vi "Get Owning Path Default Value.vi"(0 "Vector 26GHz Path Group in":refnum<class "Vector 26GHz Path Group.lvclass">, 11 "error in (no error)":errorcluster) -> (4 "Vector 26GHz Path Group out":refnum<class "Vector 26GHz Path Group.lvclass">, 6 "Path":refnum<class "Path.lvclass">, 15 "error out":errorcluster)   [LabVIEW 2023, in "RFFixtureCharact.RMM.lvlib" / "Vector 26GHz Path Group.lvclass"]
uses:
  Vector 26GHz Path Group.lvclass
  Common/Base Classes/Path/Path.lvclass
  Paths/Vector Path/Vector 26GHz Path.lvclass
  Vector 26GHz Path Group.lvclass/Vector 26GHz Path Group.ctl
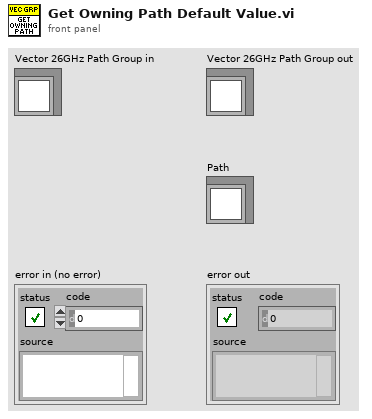
[diagram p1: front panel]
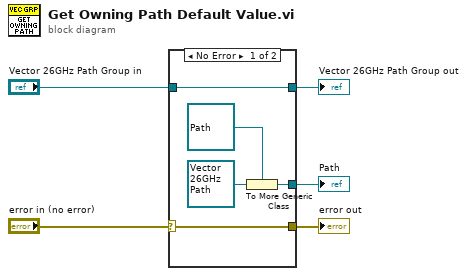
[diagram p0: block diagram]
diagram:
  n1 = case shown="No Error" "error in (no error)" {
    selector: "error in (no error)" -> [w8 w12]
    tunnel: [w9 _] -> w3
    tunnel: [w8 w12] -> w1
    tunnel: [w7 w11] -> w4
    tunnel: "Vector 26GHz Path Group in" -> [w7 w11]
    frame No Error {
      n2 = To More Generic Class(target class=refnum<class "Path.lvclass"> refnum ("Path"), reference=refnum<class "Vector 26GHz Path.lvclass"> refnum ("STS Vector Fixture Charact.lvlib:Vector Path.lvclass")) -> (generic class reference=w9:refnum<class "Path.lvclass">)
    }
    frame Error {
    }
  }
  "error out" <- w1
  "Vector 26GHz Path Group out" <- w4
  "Path" <- w3
